vi "Settings_IHS_load.vi"(8 "error in":errorcluster, 10 "Data IN":T1={"Core"={"Current VI Reference"=refnum, "Close Panel on Exit?"=FALSE, "Start Timestmap"="", "Status His"="", "Active"=FALSE, "Exit"=FALSE, "Assignment structure"="(Ta,To,X,Y,Z,0,0,O)"}, "Sample ID"="", "Cam"={"Cam"="", "Connected"=FALSE, "Sim Image"=FALSE, "Save pictures"=FALSE}, "UR"={"PC_IP"="192.168.0.15", "Remote port"=30002, "UR_IP"="192.168.0.10", "connection ID"=refnum, "Connected"=FALSE, "Sim UR signal"=FALSE, "UR Ready"=FALSE, "Ready fail"=0.0}, "Sample data"={"Insects taken from current picture"=0, "Number of insects in pick-up area"=0, "Object data"={"Object CoM X"=0.0, "Object CoM Y"=0.0, "Corrected Object orientation"=0.0, "Object length"=0.0, "Z, Height"=0.0}, "Raw Particle Measurements"=[], "Insect-data-array"=[], "Sorted Particle Measurements"=[], "Insects to pick this round"=0, "Picking array"=[], "Pixels Measurements"=[], "Tool1 to pick"=0}, "Images"={"Image"=refnum, "Image Timestamp"="", "Boarder Image"=refnum, "Vision A. Image"=refnum}, "Reshake"=0, "Settings"={"Number to try and pick"=8, "Last few"=4, "Z_Zero"=0.0, "Tool switch size"=2.0, "X-Zero"=35.0, "Y-Zero"=-406.0, "Small or XL"=12.0, "Tool1-Height"=12.0, "Tool2-Height"=12.0, "Ignore small"=12.0, "Time to Whait"=25.0}, "Assignment"={"Executing Assignment"="", "Task"="", "Tool"="", "Specimen to pick"=0, "GO"=FALSE}, "Return reason"=""} {"Sample data"."Object data"."Z, Height" format="%#_13g"}) -> (0 "error out":errorcluster, 2 "Data OUT":T1={"Core"={"Current VI Reference"=refnum, "Close Panel on Exit?"=FALSE, "Start Timestmap"="", "Status His"="", "Active"=FALSE, "Exit"=FALSE, "Assignment structure"=""}, "Sample ID"="", "Cam"={"Cam"="", "Connected"=FALSE, "Sim Image"=FALSE, "Save pictures"=FALSE}, "UR"={"PC_IP"="192.168.0.15", "Remote port"=30002, "UR_IP"="192.168.0.10", "connection ID"=refnum, "Connected"=FALSE, "Sim UR signal"=FALSE, "UR Ready"=FALSE, "Ready fail"=0.0}, "Sample data"={"Insects taken from current picture"=0, "Number of insects in pick-up area"=0, "Object data"={"Object CoM X"=0.0, "Object CoM Y"=0.0, "Corrected Object orientation"=0.0, "Object length"=0.0, "Z, Height"=0.0}, "Raw Particle Measurements"=[], "Insect-data-array"=[], "Sorted Particle Measurements"=[], "Insects to pick this round"=0, "Picking array"=[], "Pixels Measurements"=[], "Tool1 to pick"=0}, "Images"={"Image"=refnum, "Image Timestamp"="", "Boarder Image"=refnum, "Vision A. Image"=refnum}, "Reshake"=0, "Settings"={"Number to try and pick"=8, "Last few"=4, "Z_Zero"=0.1, "Tool switch size"=2.0, "X-Zero"=-35.0, "Y-Zero"=406.0, "Small or XL"=12.0, "Tool1-Height"=12.0, "Tool2-Height"=12.0, "Ignore small"=12.0, "Time to Whait"=25.0}, "Assignment"={"Executing Assignment"="", "Task"="", "Tool"="", "Specimen to pick"=0, "GO"=FALSE}, "Return reason"=""} {"Sample data"."Object data"."Z, Height" format="%#_13g"})   [LabVIEW 2024]
uses:
  SRS/controls/IHS_JKI.ctl
  <vilib>/userDefined/High Color/IMAQdx.ctl
  <vilib>/vision/Image Controls.llb/IMAQ Image.ctl
  <vilib>/Utility/xml.llb/Read From XML File(string).vi
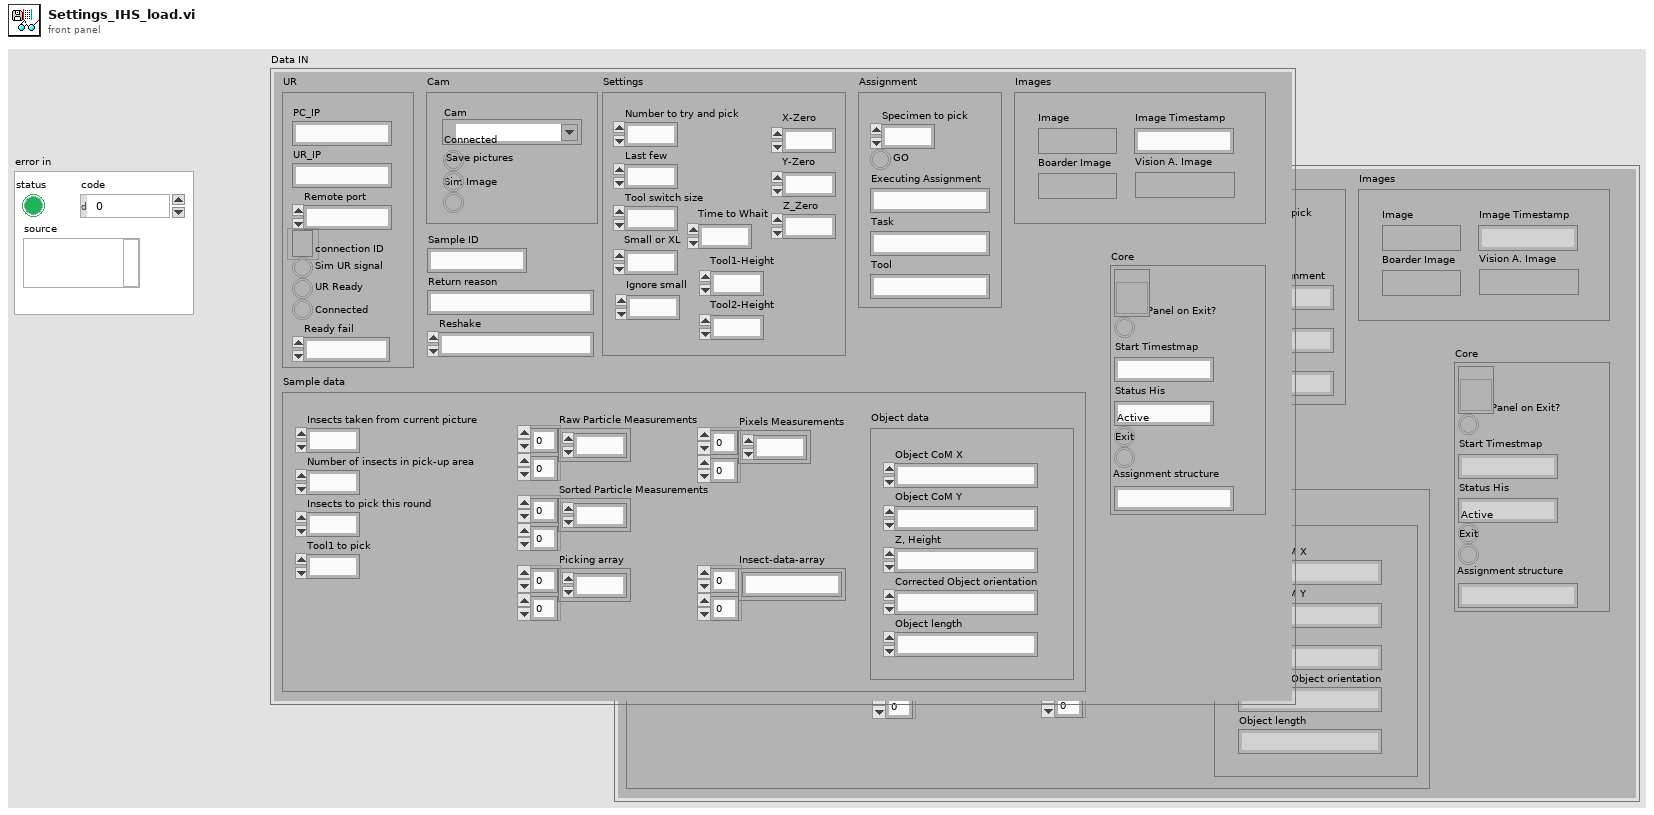
[diagram p1: front panel]
types:
  T1 = typedef "IHS_JKI.ctl" = cluster{"Core":cluster{"Current VI Reference":refnum<vi>, "Close Panel on Exit?":bool, "Start Timestmap":string, "Status His":string, "Active":bool, "Exit":bool, "Assignment structure":string}, "Sample ID":string, "Cam":cluster{"Cam":T2, "Connected":bool, "Sim Image":bool, "Save pictures":bool}, "UR":cluster{"PC_IP":string, "Remote port":u16, "UR_IP":string, "connection ID":refnum<k5>, "Connected":bool, "Sim UR signal":bool, "UR Ready":bool, "Ready fail":dbl}, "Sample data":cluster{"Insects taken from current picture":i32, "Number of insects in pick-up area":i32, "Object data":cluster{"Object CoM X":dbl, "Object CoM Y":dbl, "Corrected Object orientation":dbl, "Object length":dbl, "Z, Height":dbl}, "Raw Particle Measurements":dbl[][], "Insect-data-array":string[][], "Sorted Particle Measurements":dbl[][], "Insects to pick this round":i32, "Picking array":dbl[][], "Pixels Measurements":dbl[][], "Tool1 to pick":i32}, "Images":cluster{"Image":T3, "Image Timestamp":string, "Boarder Image":T3, "Vision A. Image":T3}, "Reshake":i32, "Settings":cluster{"Number to try and pick":i32, "Last few":i32, "Z_Zero":dbl, "Tool switch size":dbl, "X-Zero":dbl, "Y-Zero":dbl, "Small or XL":dbl, "Tool1-Height":dbl, "Tool2-Height":dbl, "Ignore small":dbl, "Time to Whait":dbl}, "Assignment":cluster{"Executing Assignment":string, "Task":string, "Tool":string, "Specimen to pick":i32, "GO":bool}, "Return reason":string}
  T2 = typedef "IMAQdx.ctl" = refnum<k21>
  T3 = typedef "IMAQ Image.ctl" = refnum<image>
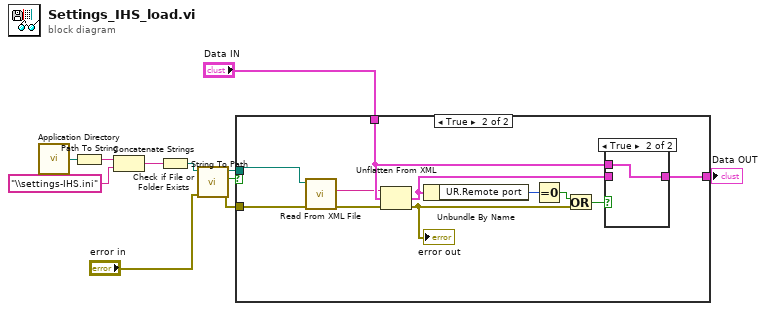
[diagram p0: block diagram]
diagram:
  n1 = call <vilib>:"Application Directory.vi"() -> ("Application Directory"=w10:path)
  n2 = Path To String(path=w10) -> (string=w11:string)
  n3 = Concatenate Strings(w11, "\\settings-IHS.ini" ("string")) -> (w8:string)
  n4 = String To Path(string=w8) -> (path=w2:path)
  n5 = call <vilib>:"Check if File or Folder Exists.vi"("error in (no error)"="error in", "path"=w2) -> ("error out"=w4:errorcluster, "file or folder exists?"=w6:bool, "dup path"=w5:path)  [unwired: 7 in]
  n6 = case shown="True" w6 {
    tunnel: w4 -> [_ w23]
    tunnel: "Data IN" -> [w12 w22]
    tunnel: [w12 w14] -> w7
    tunnel: w5 -> [_ w13]
    frame False {
    }
    frame True {
      n7 = call-poly <vilib>:"Read From XML File.vi"("error in (no error)"=w23, "XML File Path"=w13) -> ("error out"=w20:errorcluster, "XML Elements"=w21:string)  [unwired: 7 in, 1 out]
      n8 = Unflatten From XML(xml string=w21, type=w22, error in (no error)=w20) -> (value=w18:T1, error out=w15:errorcluster)
      "error out" <- w15
      n9 = Unbundle By Name(w18) -> ("UR.Remote port"=w19:u16)
      n10 = Equal To 0?(x=w19) -> (x = 0?=w17:bool)
      n11 = Or(x=w17, y=w15) -> (x .or. y?=w16:bool)
      n12 = case shown="True" w16 {
        tunnel: [w24 w25] -> w14
        tunnel: w22 -> [_ w25]
        tunnel: w18 -> [w24 _]
        frame False {
        }
        frame True {
        }
      }
    }
  }
  "Data OUT" <- w7
